vi "Control_Panel_Info.vi"() -> (1 "FMS_Color":T1)   [LabVIEW 2019]
uses:
  TypeDefs/ControlPanelColor.ctl
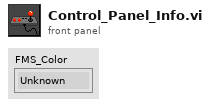
[diagram p1: front panel]
types:
  T1 = typedef "ControlPanelColor.ctl" = enum16{"Unknown", "Red", "Green", "Blue", "Yellow"}
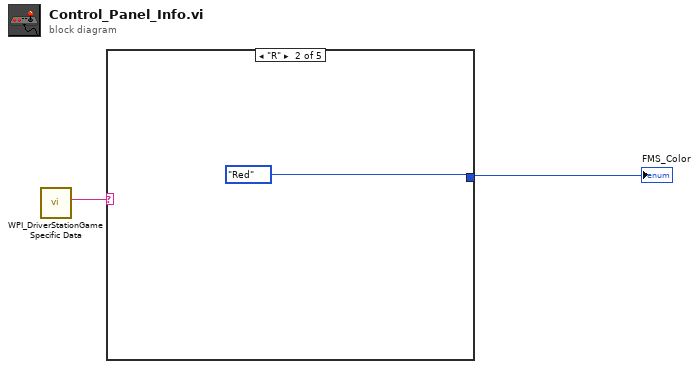
[diagram p0: block diagram]
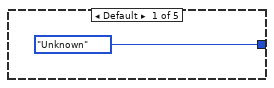
[diagram p2: hidden frame]
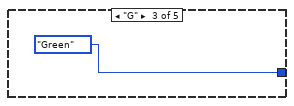
[diagram p3: hidden frame]
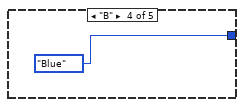
[diagram p4: hidden frame]
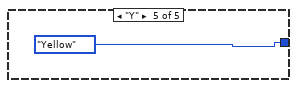
[diagram p5: hidden frame]
diagram:
  n1 = call <vilib>:"WPI_DriverStationGame Specific Data.vi"() -> ("Game Specific Data"=w2:string)  [unwired: 11 in]
  n2 = case shown="\"R\"" w2 {
    tunnel: [ControlPanelColor."Unknown" ControlPanelColor."Red" ControlPanelColor."Green" ControlPanelColor."Blue" ControlPanelColor."Yellow"] -> w1
    frame Default {
    }
    frame "R" {
    }
    frame "G" {
    }
    frame "B" {
    }
    frame "Y" {
    }
  }
  "FMS_Color" <- w1
